vi "JPL Array.vi"(11 "Boolean":bool) -> (2 "Value":dbl, 3 "Index":dbl)   [LabVIEW 2016]
uses:
  <vilib>/functionblocks/Edge Detection/One Shot Rising with Input/One Shot Rising with Input.vi
  <vilib>/functionblocks/FB Core/FB Core.xnode
  <vilib>/functionblocks/NI_FunctionBlock Libraries.lvlib
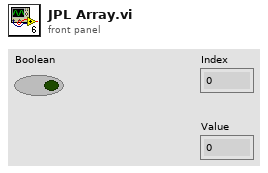
[diagram p1: front panel]
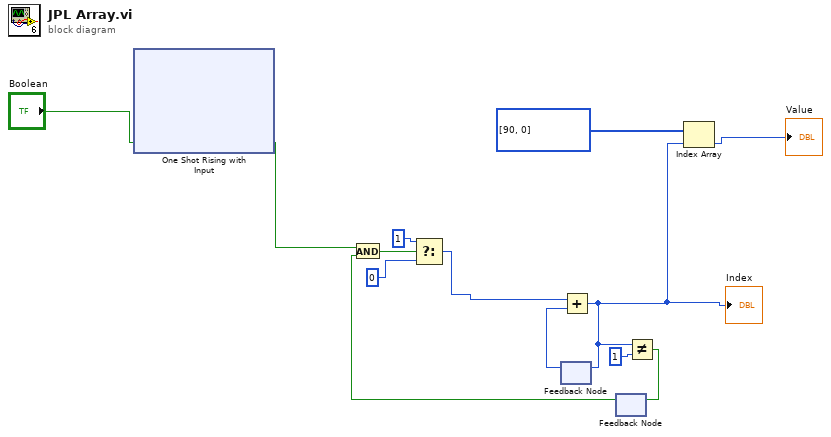
[diagram p0: block diagram]
diagram:
  n1 = xnode "One Shot Rising with Input"("input"="Boolean") -> ("output"=w2:bool)  [unwired: 1 in, 1 out]
  n2 = feedback #1() -> (w13:i32)  [unwired: 1 in]
  n3 = feedback #2() -> (w4:bool)  [unwired: 1 in]
  n4 = And(x=w2, y=w4) -> (x .and. y?=w7:bool)
  n5 = Select(t=1, s=w7, f=0) -> (s? t:f=w3:i32)
  n6 = Add(x=w3, y=w13) -> (x+y=w11:i32)
  "Index" <- w11
  n7 = feedback-in #1(w11) -> ()
  n8 = Not Equal?(x=w11, y=1) -> (x != y?=w5:bool)
  n9 = feedback-in #2(w5) -> ()
  n10 = Index Array(array=i32[] [90, 0], index=w11) -> (element=→"Value":i32)
